vi "UserinterfaceBasic.vi"() -> ()   [LabVIEW 2023]
panel:
  out "?":dbl
  in  "?":bool
  out "LED 4 (100%)":bool
  out "LED 3 (75%)":bool
  out "LED 2 (50 %)":bool
  out "LED 1 (25 %)":bool
  in  "Level":dbl(slide) scale=0.0..120.0
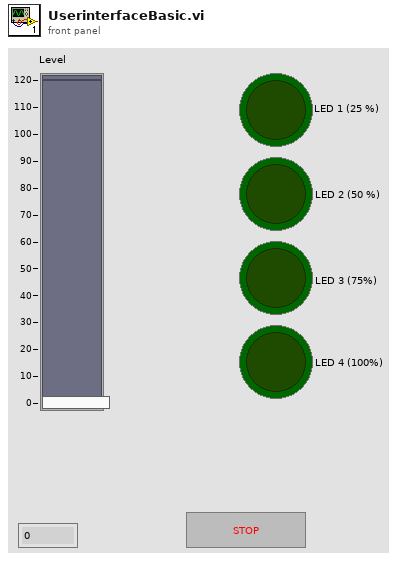
[diagram p1: front panel]
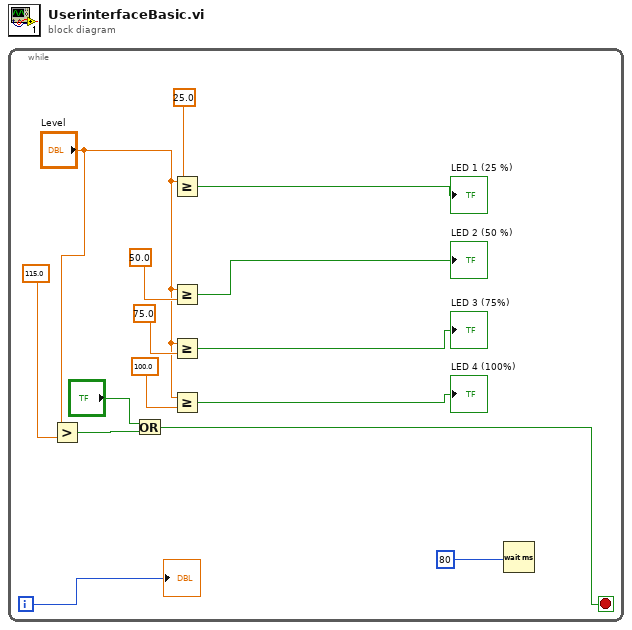
[diagram p0: block diagram]
diagram:
  n1 = while {
    i -> [w3]
    stop <- w12 stop-if-true
    n2 = Greater?(x="Level", y=115.0) -> (0:w13:bool)
    n3 = Or(x="?", y=w13) -> (x .or. y?=w12:bool)
    n4 = Greater Or Equal?(x="Level", y=25.0) -> (x >= y?=→"LED 1 (25 %)":bool)
    n5 = Greater Or Equal?(x="Level", y=50.0) -> (x >= y?=→"LED 2 (50 %)":bool)
    n6 = Greater Or Equal?(x="Level", y=75.0) -> (x >= y?=→"LED 3 (75%)":bool)
    n7 = Greater Or Equal?(x="Level", y=100.0) -> (x >= y?=→"LED 4 (100%)":bool)
    n8 = Wait (ms)(milliseconds to wait=u32 80 ("millisecond timer value")) -> ()  [unwired: 1 out]
    "?" <- w3
  }
